vi "AlazarGetMaxRecordsCapable.vi"(0 "Handle":u64, 11 "error in (no error)":errorcluster) -> (4 "Handle":u64, 6 "Samples Per Record":u32, 8 "Max Records Per Capture":u32, 10 "Return Code":u32, 15 "error out":errorcluster)   [LabVIEW 2018]
doc: "Calculate the maximum number of records that can be captured to on-board memory given the requested number of samples per record."
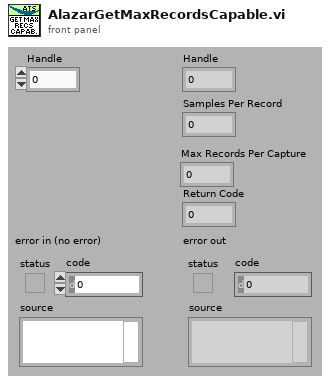
[diagram p1: front panel]
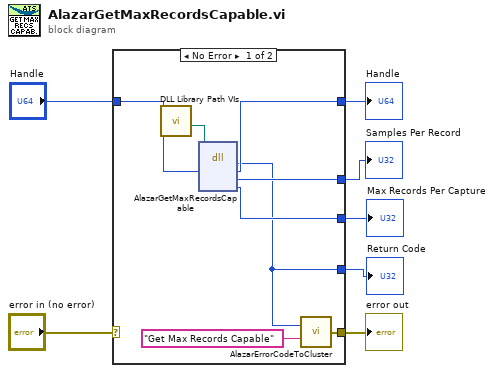
[diagram p0: block diagram]
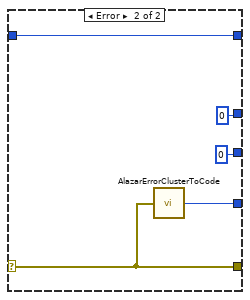
[diagram p2: hidden frame]
diagram:
  n1 = case shown="No Error" "error in (no error)" {
    selector: "error in (no error)" -> [_ w20]
    tunnel: [w11 w20] -> w6
    tunnel: [w10 w19] -> w5
    tunnel: "Handle" -> [w15 w18]
    tunnel: [w14 w18] -> w3
    tunnel: [w13 u32 0] -> w2
    tunnel: [w12 u32 0] -> w1
    frame No Error {
      n2 = call "DLL Library Path VIs.vi"() -> ("Alazar"=w8:path)  [unwired: 9 in, 2 out]
      n3 = dll-call lib="C:/Project/SerialSectOCT - FFT GPU/SerialSectOCT/Labview Software/DLL/ATSApi.dll" fn="AlazarGetMaxRecordsCapable"(path in=w8, "handle"=w15) -> ("return type"=w10:u32, "handle"=w14:u64, "samplesPerRecord"=w13:u32, "maxRecordsPerCapture"=w12:u32)  [unwired: 4 in, 2 out]
      n4 = call "AlazarErrorCodeToCluster.vi"("Message"="Get Max Records Capable", "Error Code"=w10) -> ("error out"=w11:errorcluster)
    }
    frame Error {
      n5 = call "AlazarErrorClusterToCode.vi"("error in (no error)"=w20) -> ("Error Code"=w19:u32)
    }
  }
  "Handle" <- w3
  "error out" <- w6
  "Return Code" <- w5
  "Samples Per Record" <- w2
  "Max Records Per Capture" <- w1
